vi "ReverseString.vi"(0 "InString":string) -> (1 "OutString":string)   [LabVIEW 2013]
panel:
  out "ReverseString":string
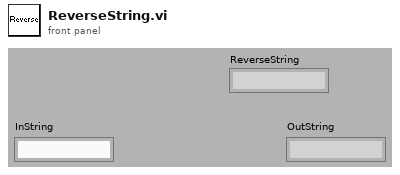
[diagram p1: front panel]
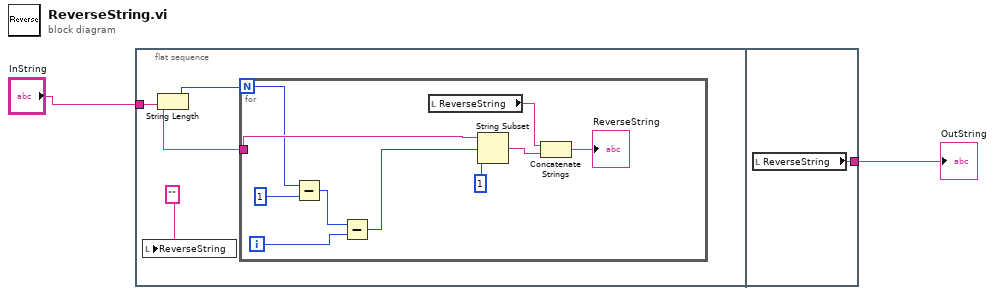
[diagram p0: block diagram]
diagram:
  n1 = flat-sequence {
    tunnel: "InString" -> [w3]
    tunnel: [w16] -> w1
    frame #0 {
      n2 = local write "ReverseString"("" ("ReverseString")) -> ()
      n3 = String Length(string=w3) -> (length=w4:i32)
      n4 = for {
        N: w4 -> [w13]
        tunnel: w3 -> [w15]
        i -> [w14]
        n5 = Subtract(x=w13, y=1) -> (x-y=w11:i32)
        n6 = Subtract(x=w11, y=w14) -> (x-y=w6:i32)
        n7 = local read "ReverseString"() -> (w7:string)
        n8 = String Subset(string=w15, offset (0)=w6, length (rest)=1 ("length (rest)")) -> (substring=w9:string)
        n9 = Concatenate Strings(w7, w9) -> (→"ReverseString":string)
      }
    }
    frame #1 {
      n10 = local read "ReverseString"() -> (w16:string)
    }
  }
  "OutString" <- w1
